vi "Caraya Verify Hello Caraya.vi"(8 "error in (no error)":errorcluster) -> (0 "error out":errorcluster)   [LabVIEW 2020, in "Caraya Extension Test Suite.lvclass"]
uses:
  Caraya Extension Test Suite.lvclass
  Caraya Extension Test Suite.lvclass/Caraya Extension Test Suite.ctl
  Caraya.Extension/Caraya.Extension.lvlib
  <vilib>/addons/_JKI Toolkits/Caraya/classes/Test/Test.lvclass
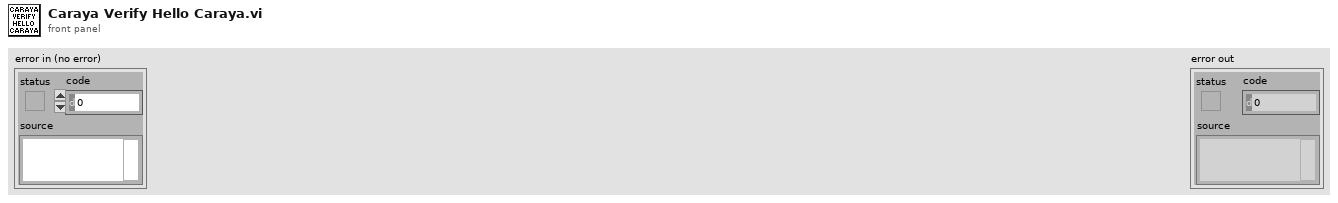
[diagram p1: front panel]
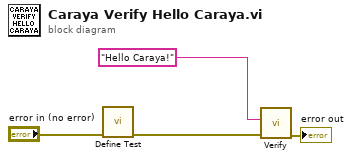
[diagram p0: block diagram]
diagram:
  n1 = call <vilib>:"Define Test.vi"("error in (no error)"="error in (no error)") -> ("error out"=w3:errorcluster)  [unwired: 9 in, 1 out]
  n2 = call "Verify.vi"("error in"=w3, "Test Data"="Hello Caraya!") -> ("error out"=→"error out":errorcluster)  [unwired: 9 in]
